vi "Send Error.vi"(8 "error in (no error)":errorcluster, 10 "Message":string, 11 "Build Events API in":refnum<class "Build Events API.lvclass">) -> (0 "error out":errorcluster, 3 "Build Events API out":refnum<class "Build Events API.lvclass">)   [LabVIEW 2020, in "Builder Tools.lvlib" / "Build Events API.lvclass"]
uses:
  Build Events API.lvclass
  Build Events API.lvclass/Build Events API.ctl
  Error Data.ctl
  Builder Tools.lvlib
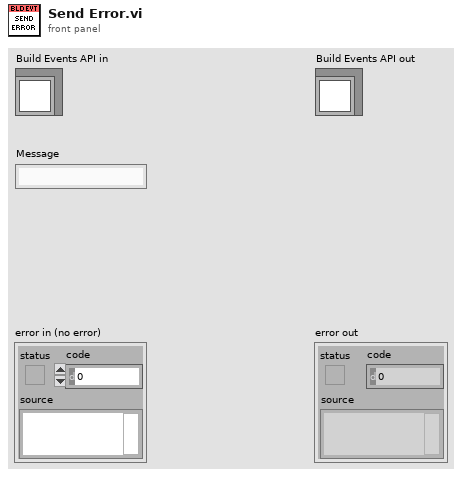
[diagram p1: front panel]
types:
  T1 = typedef "Builder Tools.lvlib/Error Data.ctl" = cluster{"Message":string}
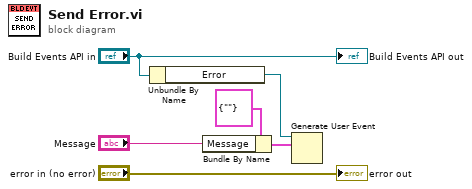
[diagram p0: block diagram]
diagram:
  n1 = Unbundle By Name("Build Events API in") -> ("Error"=w4:refnum<user-event>)
  n2 = Bundle By Name(cluster=T1 {"Message"=""} ("event data"), "Message"="Message") -> (w2:T1)
  n3 = Generate User Event(user event=w4, event data cluster=w2) -> ()  [unwired: 2 in, 2 out]
  "error out" <- "error in (no error)"
  "Build Events API out" <- "Build Events API in"
